vi "plant_stop.vi"(0 "Dataflow In":errorcluster, 1 "Stop In":refnum<vi>) -> (2 "Stop Out":bool, 5 "Dataflow Out":errorcluster)   [LabVIEW 2019]
uses:
  lib/libSimulationControl/libSimulationControl.lvlib
panel:
  # "*******************************************************************\nBiogas Plant Control\n\nAuthor: Paul Zügel\nGCSC-Frankfurt am Main 2020\n\n*******************************************************************"
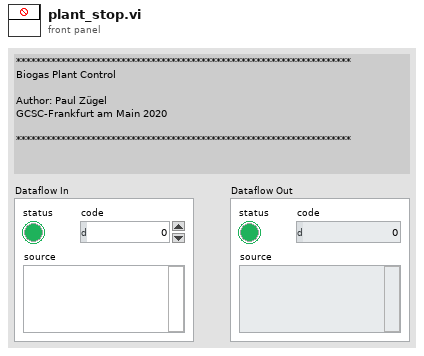
[diagram p1: front panel]
types:
  T1 = enum32{"Invalid", "Standard", "Closed", "Hidden", "Minimized", "Maximized"}
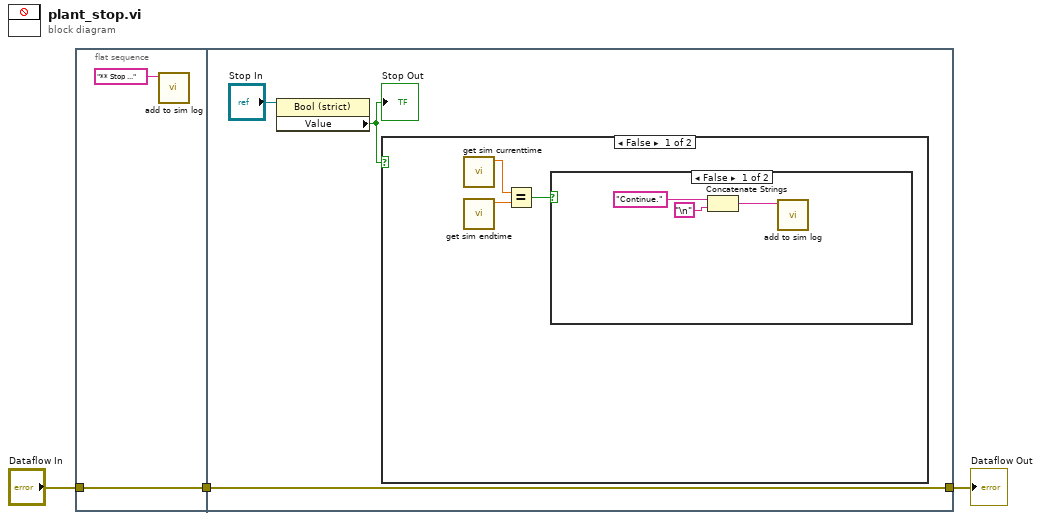
[diagram p0: block diagram]
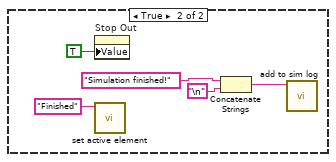
[diagram p2: hidden frame]
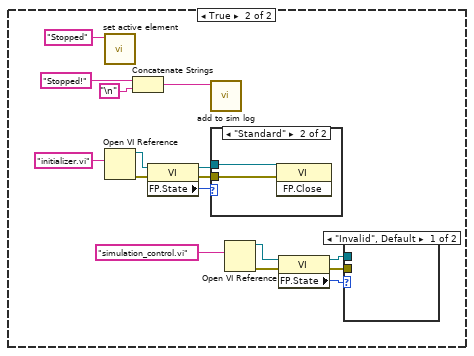
[diagram p3: hidden frame]
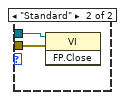
[diagram p5: hidden frame]
diagram:
  n1 = flat-sequence {
    tunnel: "Dataflow In" -> [w5]
    tunnel: [w5] -> w2
    tunnel: w2 -> [w8]
    tunnel: [w8] -> w1
    frame #0 {
      n2 = call "add to sim log.vi"("log"="** Stop ..." ("string")) -> ()  [unwired: 10 in, 1 out]
    }
    frame #1 {
      n3 = property on="Property Node" class="Bool (strict)"(reference="Stop In") -> ("Value"=w7:bool)  [unwired: 1 in, 2 out]
      "Stop Out" <- w7
      n4 = case shown="False" w7 {
        frame False {
          n5 = call "get sim currenttime.vi"() -> ("function return"=w9:dbl)  [unwired: 10 in, 1 out]
          n6 = call "get sim endtime.vi"() -> ("function return"=w10:dbl)  [unwired: 10 in, 1 out]
          n7 = Equal?(x=w9, y=w10) -> (x = y?=w11:bool)
          n8 = case shown="False" w11 {
            frame False {
              n9 = Concatenate Strings("Continue." ("string"), "\n") -> (w14:string)
              n10 = call "add to sim log.vi"("log"=w14) -> ()  [unwired: 10 in, 1 out]
            }
            frame True {
              n11 = property on="Stop Out" class="Bool (strict)"("Value"=TRUE ("Stop Button")) -> ()  [unwired: 2 in, 2 out]
              n12 = call "set active element.vi"("elem"="Finished") -> ()  [unwired: 10 in, 1 out]
              n13 = Concatenate Strings("Simulation finished!" ("log"), "\n") -> (w16:string)
              n14 = call "add to sim log.vi"("log"=w16) -> ()  [unwired: 10 in, 1 out]
            }
          }
        }
        frame True {
          n15 = call "set active element.vi"("elem"="Stopped") -> ()  [unwired: 10 in, 1 out]
          n16 = Open VI Reference(vi path="initializer.vi") -> (vi reference=w25:refnum<vi>, error out=w24:errorcluster)  [unwired: 5 in]
          n17 = Concatenate Strings("Stopped!" ("string"), "\n") -> (w20:string)
          n18 = property class="VI"(reference=w25, error in=w24) -> (reference out=w27:refnum<vi>, error out=w26:errorcluster, "FP.State"=w28:T1)
          n19 = call "add to sim log.vi"("log"=w20) -> ()  [unwired: 10 in, 1 out]
          n20 = case shown="\"Standard\"" w28 {
            tunnel: w27 -> [_ w37]
            tunnel: w26 -> [_ w36]
            frame "Invalid", Default {
            }
            frame "Standard" {
              n21 = invoke class="VI" method="FP.Close"(reference=w37, error in=w36) -> ()  [unwired: 1 in, 3 out]
            }
          }
          n22 = Open VI Reference(vi path="simulation_control.vi") -> (vi reference=w30:refnum<vi>, error out=w29:errorcluster)  [unwired: 5 in]
          n23 = property class="VI"(reference=w30, error in=w29) -> (reference out=w32:refnum<vi>, error out=w31:errorcluster, "FP.State"=w33:T1)
          n24 = case shown="\"Invalid\", Default" w33 {
            tunnel: w32 -> [_ w39]
            tunnel: w31 -> [_ w38]
            frame "Invalid", Default {
            }
            frame "Standard" {
              n25 = invoke class="VI" method="FP.Close"(reference=w39, error in=w38) -> ()  [unwired: 1 in, 3 out]
            }
          }
        }
      }
    }
  }
  "Dataflow Out" <- w1
